vi "semester_1_project_client.vi"() -> ()   [LabVIEW 2024]
uses:
  semester_1_project_global.vi
panel:
  in  "stop":bool
  in  "Sample Rate":dbl=100.0
  out "Humidity Average":dbl
  out "Temperature Average":dbl
  out "Humidity":dbl
  out "Temperature":dbl
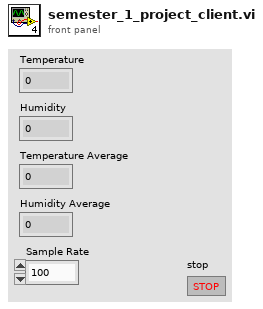
[diagram p1: front panel]
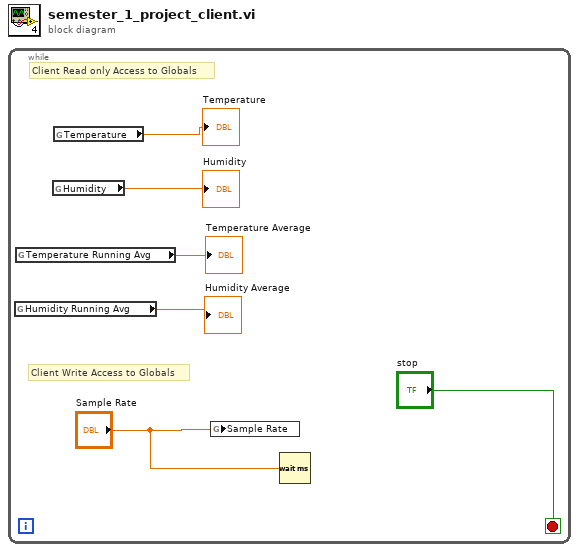
[diagram p0: block diagram]
diagram:
  n1 = while {
    stop <- "stop" stop-if-true
    # "Client Write Access to Globals"
    # "Client Read only Access to Globals"
    n2 = global read "semester_1_project_global.vi" "Humidity Running Avg"() -> (→"Humidity Average":dbl)
    n3 = global read "semester_1_project_global.vi" "Temperature Running Avg"() -> (→"Temperature Average":dbl)
    n4 = global read "semester_1_project_global.vi" "Humidity"() -> (→"Humidity":dbl)
    n5 = global read "semester_1_project_global.vi" "Temperature"() -> (→"Temperature":dbl)
    n6 = global write "semester_1_project_global.vi" "Sample Rate"("Sample Rate") -> ()
    n7 = Wait (ms)(milliseconds to wait="Sample Rate") -> ()  [unwired: 1 out]
  }
